vi "CAEN_CUR_MON (SubVI).vi"(8 "error in (no error)":errorcluster, 11 "Cluster in":T1={"BAUDE RATE"=enum."9600", "VISA RESOURCE NAME"=""}) -> (0 "error out":errorcluster, 3 "DBL out":dbl[](array[numeric]))   [LabVIEW 2020]
uses:
  Desktop/eTPC/subVIs for MKS/INITIALIZATION PFEIFFER.ctl
  <vilib>/Instr/_visa.llb/VISA Configure Serial Port (Instr).vi
  <instrlib>/PV ActiveLine/PV ActiveLine.lvlib
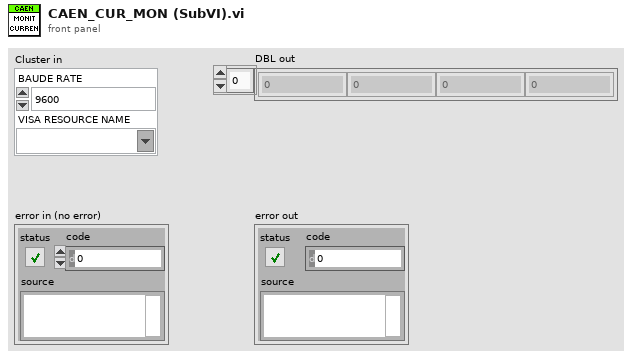
[diagram p1: front panel]
types:
  T1 = typedef "INITIALIZATION PFEIFFER.ctl" = cluster{"BAUDE RATE":enum32{"38400", "19200", "9600", "4800"}, "VISA RESOURCE NAME":refnum<visa-resource-name>}
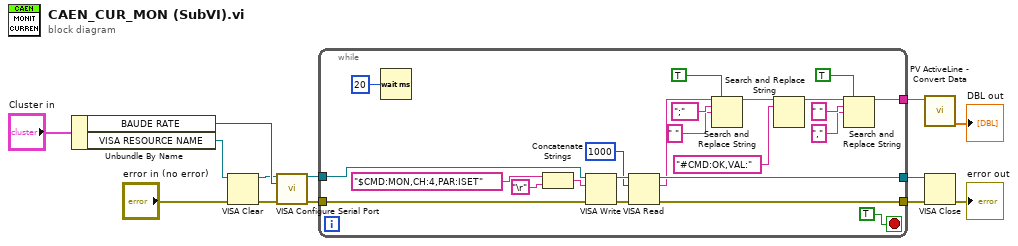
[diagram p0: block diagram]
diagram:
  n1 = Unbundle By Name("Cluster in") -> ("BAUDE RATE"=w11:enum32{"38400", "19200", "9600", "4800"}, "VISA RESOURCE NAME"=w1:refnum<visa-resource-name>)
  n2 = VISA Clear(VISA resource name=w1, error in (no error)="error in (no error)") -> (VISA resource name out=w5:refnum<visa-resource-name>, error out=w4:errorcluster)
  n3 = call-poly "VISA Configure Serial Port"("VISA resource name"=w5, "baud rate (9600)"=w11, "error in (no error)"=w4) -> ("VISA resource name out"=w9:refnum<visa-resource-name>, "error out"=w10:errorcluster)  [unwired: 11 in]
  n4 = while {
    tunnel: w9 -> [w36]
    tunnel: w10 -> [w35]
    tunnel: [w29] -> w12
    tunnel: [w28] -> w13
    tunnel: [w15] -> w6
    stop <- TRUE stop-if-true
    n5 = Wait (ms)(milliseconds to wait=u32 20) -> ()  [unwired: 1 out]
    n6 = Concatenate Strings("$CMD:MON,CH:4,PAR:ISET" ("string"), "\r") -> (w26:string)
    n7 = VISA Write(VISA resource name=w36, write buffer=w26, error in (no error)=w35) -> (VISA resource name out=w31:refnum<visa-resource-name>, error out=w30:errorcluster)  [unwired: 1 out]
    n8 = VISA Read(VISA resource name=w31, byte count=u32 1000, error in (no error)=w30) -> (VISA resource name out=w28:refnum<visa-resource-name>, read buffer=w24:string, error out=w29:errorcluster)  [unwired: 1 out]
    n9 = Search and Replace String(replace all?=TRUE ("replace all? (F)"), input string=w24, search string=";", replace string=" " ("replace string (\"\")")) -> (result string=w19:string)  [unwired: 4 in, 3 out]
    n10 = Search and Replace String(input string=w19, search string="#CMD:OK,VAL:") -> (result string=w14:string)  [unwired: 6 in, 3 out]
    n11 = Search and Replace String(replace all?=TRUE ("replace all? (F)"), input string=w14, search string=" ", replace string="," ("replace string (\"\")")) -> (result string=w15:string)  [unwired: 4 in, 3 out]
  }
  n12 = call <instrlib>:"PV ActiveLine - Convert Data.vi"("String in"=w6) -> ("DBL out"=→"DBL out":dbl[])  [unwired: 7 in, 3 out]
  n13 = VISA Close(VISA resource name=w13, error in (no error)=w12) -> (error out=→"error out":errorcluster)
